vi "Extract topology based controls.vi"(8 "error in":errorcluster, 11 "SwitchMatrix in":refnum<class "SwitchMatrix.lvclass">) -> (0 "error out":errorcluster, 3 "SwitchMatrix out":refnum<class "SwitchMatrix.lvclass">)   [LabVIEW 2019, in "SwitchMatrix.lvlib" / "SwitchMatrix.lvclass"]
uses:
  Library/SwitchMatrix.lvclass
  Library/SwitchMatrix.lvclass/SwitchMatrix.ctl
  <vilib>/regexp/Match Regular Expression.xnode
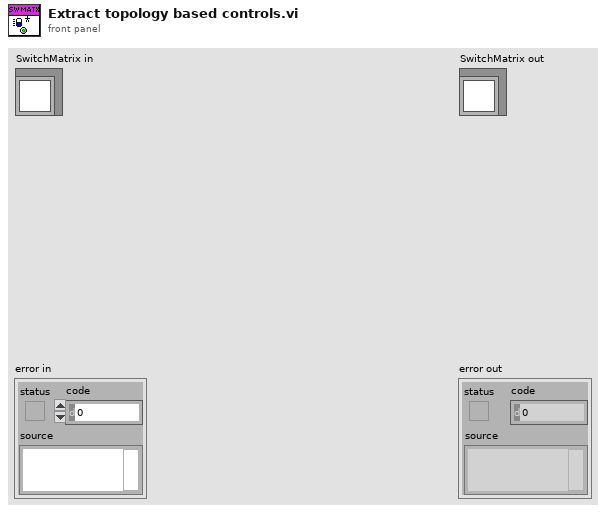
[diagram p1: front panel]
types:
  T1 = typedef "SwitchMatrix.lvlib/SwitchMatrix.lvclass/Topology_Mode.ctl" = enum16{"Single", "Dual", "Quad", "Octal", "Sixteen"}
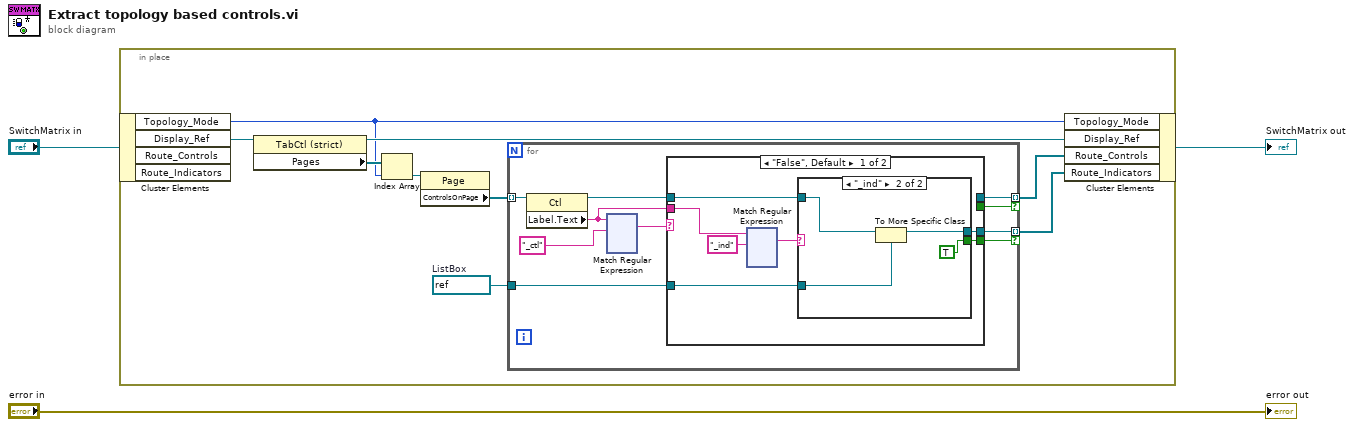
[diagram p0: block diagram]
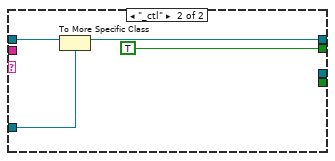
[diagram p3: hidden frame]
diagram:
  n1 = in-place {
    w4 = refnum<vi> refnum  # ListBox
    n2 = in-place-cluster #1("SwitchMatrix in") -> ("Topology_Mode"=w9:T1, "Display_Ref"=w12:refnum<vi>)  [unwired: 2 out]
    n3 = property class="TabCtl (strict)"(reference=w12) -> (reference out=w11:refnum<vi>, "Pages"=w10:refnum<vi>[])  [unwired: 1 in, 1 out]
    n4 = Index Array(array=w10, index=w9) -> (element=w8:refnum<vi>)
    n5 = property class="Page"(reference=w8) -> ("ControlsOnPage"=w7:refnum<vi>[])  [unwired: 1 in, 2 out]
    n6 = for {
      tunnel: w7 -> [w22] mode=indexing
      tunnel: [w18] -> w6 mode=indexing if=w17
      tunnel: [w16] -> w5 mode=indexing if=w15
      tunnel: w4 -> [w14]
      n7 = property class="Ctl"(reference=w22) -> (reference out=w19:refnum<vi>, "Label.Text"=w13:string)  [unwired: 1 in, 1 out]
      n8 = xnode "Match Regular Expression"("input string"=w13, "regular expression"="_ctl") -> ("whole match"=w20:string)  [unwired: 4 in, 4 out]
      n9 = case shown="\"False\", Default" w20 {
        tunnel: w19 -> [w26 w151]
        tunnel: [_ w149] -> w18
        tunnel: [_ TRUE] -> w17
        tunnel: w13 -> [w29 _]
        tunnel: [w25 _] -> w16
        tunnel: [w24 _] -> w15
        tunnel: w14 -> [w23 w148]
        frame "False", Default {
          n10 = xnode "Match Regular Expression"("input string"=w29, "regular expression"="_ind") -> ("whole match"=w27:string)  [unwired: 4 in, 4 out]
          n11 = case shown="\"_ind\"" w27 {
            tunnel: w26 -> [_ w32]
            tunnel: [_ w31] -> w25
            tunnel: [_ TRUE] -> w24
            tunnel: w23 -> [_ w30]
            frame "False", Default {
            }
            frame "_ind" {
              n12 = To More Specific Class(target class=w30, reference=w32) -> (specific class reference=w31:refnum<vi>)  [unwired: 1 in, 1 out]
            }
          }
        }
        frame "_ctl" {
          n13 = To More Specific Class(target class=w148, reference=w151) -> (specific class reference=w149:refnum<vi>)  [unwired: 1 in, 1 out]
        }
      }
    }
    n14 = in-place-cluster #1("Topology_Mode"=w9, "Display_Ref"=w11, "Route_Controls"=w6, "Route_Indicators"=w5) -> (→"SwitchMatrix out":refnum<class "SwitchMatrix.lvclass">)
  }
  "error out" <- "error in"
